vi "AddTestMethod_Item_OnCommand.vi"(10 "Command ID":string, 11 "Object":T1) -> ()   [LabVIEW 2013]
uses:
  <resource>/Framework/Providers/API/ItemRef.ctl
panel:
  out "error out":errorcluster
  in  "error in":errorcluster
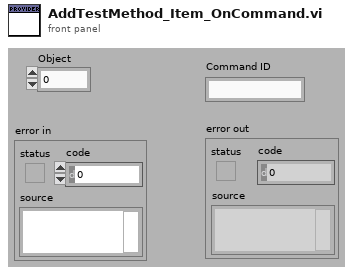
[diagram p1: front panel]
types:
  T1 = typedef "ItemRef.ctl" = u64
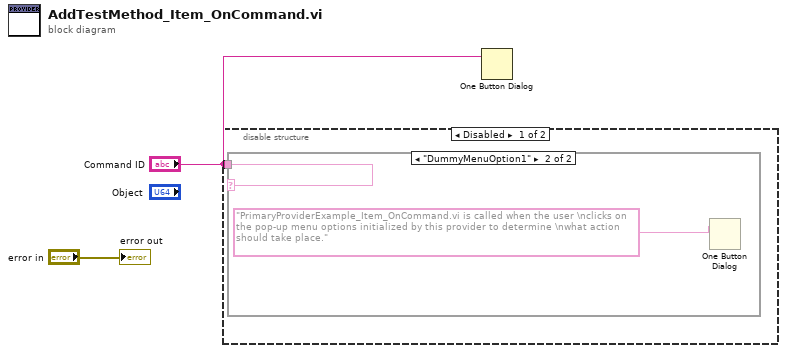
[diagram p0: block diagram]
diagram:
  n1 = disable-structure shown="Disabled" {
    disable-tunnel: "Command ID" -> [w3 _]
    frame Disabled {
      n2 = case shown="\"DummyMenuOption1\"" w3 {
        frame Default {
        }
        frame "DummyMenuOption1" {
          n3 = One Button Dialog(message="PrimaryProviderExample_Item_OnCommand.vi is called when the user \nclicks on the pop-up menu options initialized by this provider to determine \nwhat action should take place.") -> ()  [unwired: 1 in, 1 out]
        }
      }
    }
    frame Enabled {
    }
  }
  n4 = One Button Dialog(message="Command ID") -> ()  [unwired: 1 in, 1 out]
  "error out" <- "error in"
